vi "params.vi"(8 "error in (no error)":errorcluster, 11 "dataTA in":refnum<class "dataTA.lvclass">) -> (0 "error out":errorcluster, 3 "dataTA out":refnum<class "dataTA.lvclass">)   [LabVIEW 2019, in "dataTA.lvlib" / "dataTA.lvclass"]
uses:
  dataTA.lvclass
  D:/github/TransientAbsorptionDAQ.lv/_data/_data.lvlibp/_dataClass/_data.lvclass
  dataTA.lvclass/dataTA.ctl
  <vilib>/Analysis/NI_AALBase.lvlib
panel:
  in  "reset accum.":bool
  in  "Scale.Range:Maximum":dbl(slide)=3.2550885998350587 caption="diff scale range" scale=1.0..1000.0
  in  "trig2 level":dbl(slide)=1587.9396984924624 scale=0.0..2000.0
  out "Tank 2":dbl(slide) scale=0.0..2000.0
  out "Tank 2 - std":dbl(slide) scale=0.0..2000.0
  out "Tank 2 + std":dbl(slide) scale=0.0..2000.0
  in  "use dynamic offset?":bool
  in  "camera max scale":u16(ring)=1 items=["12-bit", "14-bit", "16-bit"]
  in  "trig1 level":dbl(slide)=783.9195979899498 scale=0.0..2000.0
  out "Tank 1":dbl(slide)=552.7638190954774 scale=0.0..2000.0
  out "Tank 1 - std":dbl(slide) scale=0.0..2000.0
  out "Tank 1 + std":dbl(slide) scale=0.0..2000.0
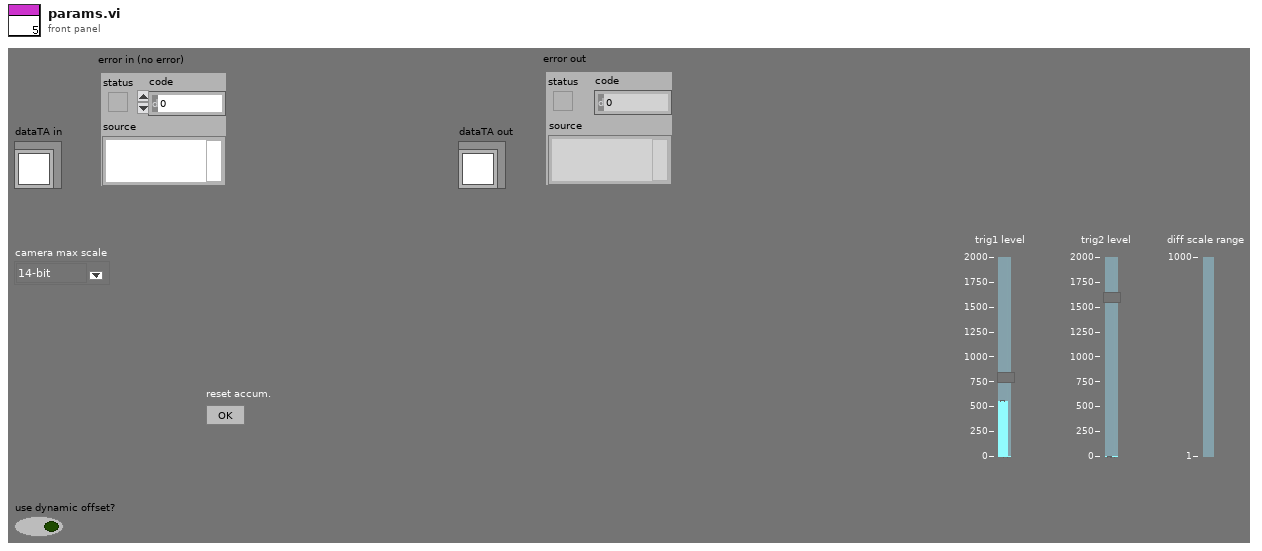
[diagram p1: front panel]
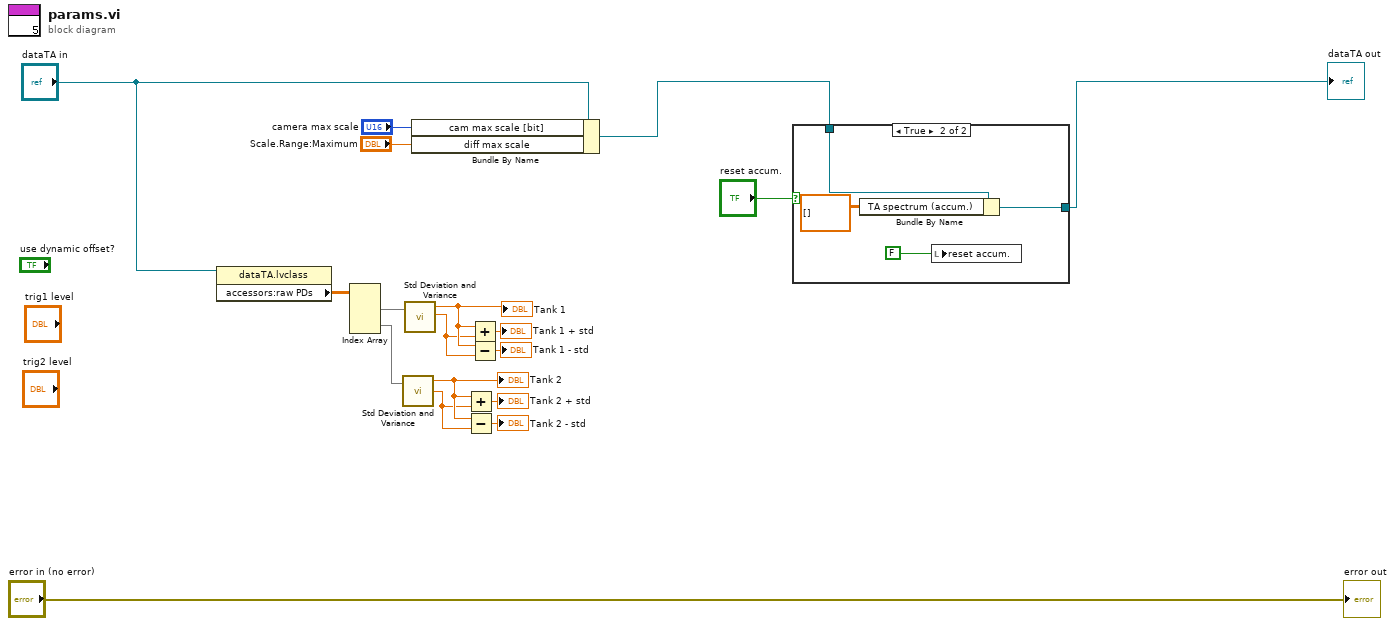
[diagram p0: block diagram]
diagram:
  n1 = property class="dataTA.lvclass"(reference="dataTA in") -> ("accessors:raw PDs"=w16:dbl[][])  [unwired: 1 in, 2 out]
  n2 = Index Array(array=w16) -> (element #1=w15:dbl[], element #2=w12:dbl[])  [unwired: 4 in]
  n3 = call <vilib>:"Std Deviation and Variance.vi"("X"=w12) -> ("mean"=w11:dbl, "standard deviation"=w10:dbl)  [unwired: 1 in, 1 out]
  "Tank 2" <- w11
  n4 = call <vilib>:"Std Deviation and Variance.vi"("X"=w15) -> ("mean"=w7:dbl, "standard deviation"=w6:dbl)  [unwired: 1 in, 1 out]
  "Tank 1" <- w7
  n5 = Bundle By Name(cluster="dataTA in", "cam max scale [bit]"="camera max scale", "diff max scale"="Scale.Range:Maximum") -> (w2:refnum<class "dataTA.lvclass">)
  n6 = Add(x=w11, y=w10) -> (x+y=→"Tank 2 + std":dbl)
  n7 = Subtract(x=w11, y=w10) -> (x-y=→"Tank 2 - std":dbl)
  n8 = Add(x=w7, y=w6) -> (x+y=→"Tank 1 + std":dbl)
  n9 = Subtract(x=w7, y=w6) -> (x-y=→"Tank 1 - std":dbl)
  n10 = case shown="True" "reset accum." {
    tunnel: w2 -> [w19 w23]
    tunnel: [w19 w21] -> w1
    frame False {
    }
    frame True {
      n11 = Bundle By Name(cluster=w23, "TA spectrum (accum.)"=dbl[][] []) -> (w21:refnum<class "dataTA.lvclass">)
      n12 = local write "reset accum."(FALSE) -> ()
    }
  }
  "dataTA out" <- w1
  "error out" <- "error in (no error)"
